vi "Add Widget to Container.vi"(5 "Container":refnum<class "QWidget.lvclass">, 8 "Error In":errorcluster, 9 "Label":string, 10 "Widget":refnum<class "QWidget.lvclass">, 11 "Abstract Widget Builder in":refnum<class "Abstract Widget Builder.lvclass">) -> (0 "Error Out":errorcluster, 3 "Abstract Widget Builder out":refnum<class "Abstract Widget Builder.lvclass">)   [LabVIEW 2013, in "Abstract Widget Builder.lvclass"]
uses:
  Abstract Widget Builder.lvclass
  src/LabVIEW/Qt Widgets/QWidget/QWidget.lvclass
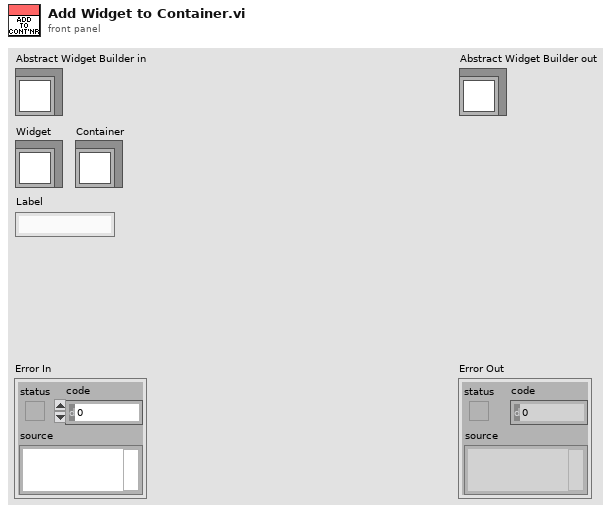
[diagram p1: front panel]
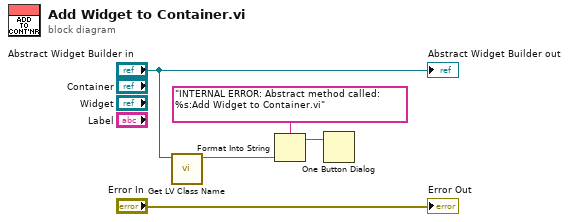
[diagram p0: block diagram]
diagram:
  n1 = call <vilib>:"Get LV Class Name.vi"("object"="Abstract Widget Builder in") -> ("class name"=w3:string)  [unwired: 9 in, 1 out]
  n2 = Format Into String(format string="INTERNAL ERROR: Abstract method called:  %s:Add Widget to Container.vi" ("message"), w3) -> (resulting string=w2:string)  [unwired: 2 in, 1 out]
  n3 = One Button Dialog(message=w2) -> ()  [unwired: 1 in, 1 out]
  "Error Out" <- "Error In"
  "Abstract Widget Builder out" <- "Abstract Widget Builder in"
